vi "Validate Hardware Custom Device API Version 1.vi"(8 "error in (no error)":errorcluster, 11 "Hardware Ref in":T1 format="%.0x") -> (0 "error out":errorcluster, 3 "Hardware Ref out":T1 format="%.0x")   [LabVIEW 2017, in "Routing and Faulting Hardware API.lvlib"]
uses:
  Routing and Faulting Hardware API.lvlib
  <vilib>/NI Veristand/Custom Device API/Custom Device Item Ref.ctl
  Routing and Faulting Hardware API Constants.vi
  <vilib>/NI Veristand/Custom Device API/Custom Device API.lvlib
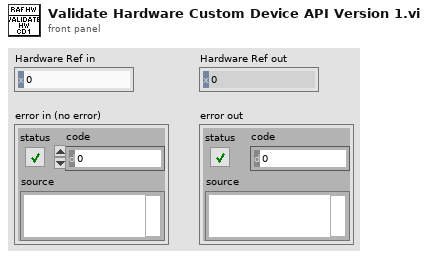
[diagram p1: front panel]
types:
  T1 = typedef "Custom Device API.lvlib/Custom Device Item Ref.ctl" = u64
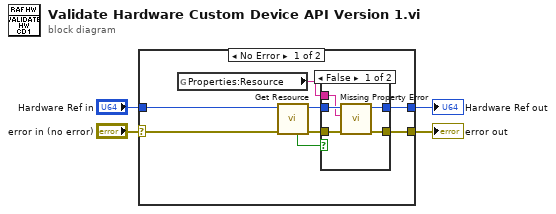
[diagram p0: block diagram]
diagram:
  n1 = case shown="No Error" "error in (no error)" {
    selector: "error in (no error)" -> [w11 w21]
    tunnel: [w9 w21] -> w2
    tunnel: [w7 w20] -> w3
    tunnel: "Hardware Ref in" -> [w12 w20]
    frame No Error {
      n2 = global read "Routing and Faulting Hardware API Constants.vi" "Properties:Resource"() -> (w5:string)
      n3 = call "Get Resource.vi"("error in (no error)"=w11, "Hardware Ref in"=w12) -> ("error out"=w10:errorcluster, "Hardware Ref out"=w8:T1, "Found?"=w6:bool)  [unwired: 6 in, 1 out]
      n4 = case shown="False" w6 {
        tunnel: w10 -> [w17 w19]
        tunnel: [w16 w19] -> w9
        tunnel: w8 -> [w15 w18]
        tunnel: [w14 w18] -> w7
        tunnel: w5 -> [w13 _]
        frame False {
          n5 = call "Missing Property Error.vi"("error in (no error)"=w17, "Property Name"=w13, "Hardware Ref in"=w15) -> ("error out"=w16:errorcluster, "Hardware Ref out"=w14:T1)  [unwired: 7 in]
        }
        frame True {
        }
      }
    }
    frame Error {
    }
  }
  "Hardware Ref out" <- w3
  "error out" <- w2
